vi "Wait For Fresh DO Signal Bank.vi"(8 "error in (no error)":errorcluster, 10 "timeout (ms)":i32=5000) -> (0 "error out":errorcluster={"status"=TRUE, "code"=555, "source"="Timed out waiting for Signal Bank."})   [LabVIEW 2020]
uses:
  PXI Globals.vi
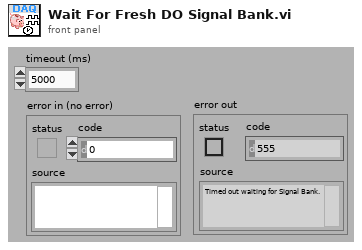
[diagram p1: front panel]
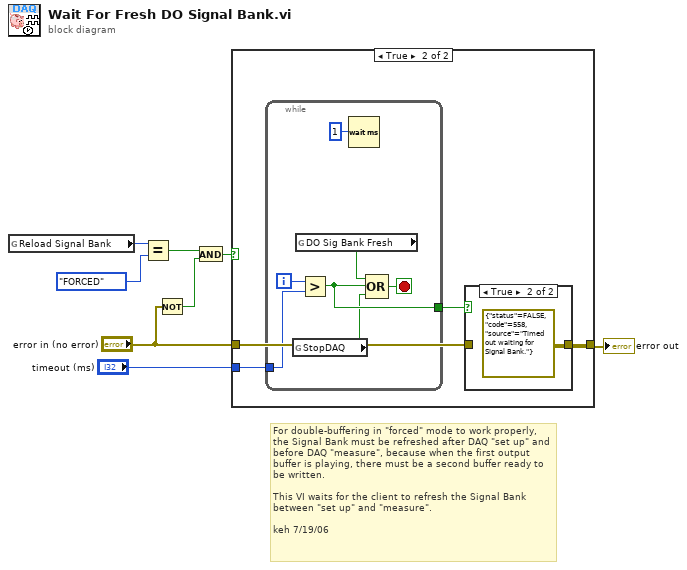
[diagram p0: block diagram]
diagram:
  # "For double-buffering in \"forced\" mode to work properly, the Signal Bank must be refreshed after DAQ \"set up\" and before DAQ \"measure\", because when the first output buffer is playing, there must be a second buffer ready to be written. \n\nThis VI waits for the client to refresh the Signal Bank between \"set up\" and \"measure\".\n\nkeh 7/19/06"
  n1 = global read "PXI Globals.vi" "Reload Signal Bank"() -> (w8:enum32{"OFF", "ENABLED", "FORCED"})
  n2 = Equal?(x=w8, y=enum16{"OFF", "ENABLED", "FORCED"}."FORCED") -> (x = y?=w2:bool)
  n3 = Not(x="error in (no error)") -> (.not. x?=w5:bool)
  n4 = And(x=w2, y=w5) -> (x .and. y?=w4:bool)
  n5 = case shown="True" w4 {
    tunnel: "error in (no error)" -> [w9 w12]
    tunnel: [w9 w11] -> w6
    tunnel: "timeout (ms)" -> [_ w10]
    frame False {
    }
    frame True {
      n6 = while {
        tunnel: w10 -> [w18]
        tunnel: [w19] -> w13
        i -> [w20]
        stop <- w21 stop-if-true
        n7 = global read "PXI Globals.vi" "StopDAQ"() -> (w17:bool)
        n8 = global read "PXI Globals.vi" "DO Sig Bank Fresh"() -> (w16:bool)
        n9 = Greater?(x=w20, y=w18) -> (0:w19:bool)
        n10 = Wait (ms)(milliseconds to wait=1) -> ()  [unwired: 1 out]
        n11 = Compound Arithmetic op=OR(w16, w19, w17) -> (w21:bool)
      }
      n12 = case shown="True" w13 {
        tunnel: w12 -> [w14 _]
        tunnel: [w14 errorcluster {"status"=FALSE, "code"=558, "source"="Timed out waiting for Signal Bank."} ("error out 2")] -> w11
        frame False {
        }
        frame True {
        }
      }
    }
  }
  "error out" <- w6
